vi "requestStatus.vi"(8 "error in (no error)":errorcluster, 11 "MonoClientCommunicator in":refnum<class "MonoClientCommunicator.lvclass">) -> (0 "error out":errorcluster, 2 "DeviceStatus":T1, 3 "MonoClientCommunicator out":refnum<class "MonoClientCommunicator.lvclass">)   [LabVIEW 2016, in "MonoClientCommunicator.lvclass"]
uses:
  MonoClientCommunicator.lvclass
  Typedefs/DeviceStatus.ctl
  Typedefs/MonoCommand.ctl
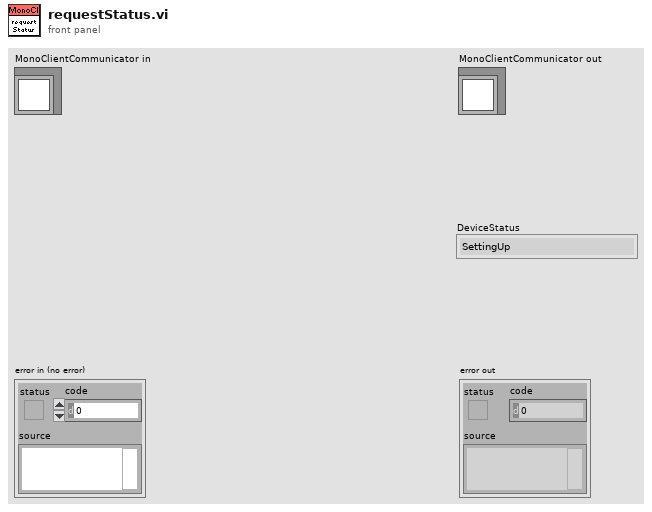
[diagram p1: front panel]
types:
  T1 = typedef "DeviceStatus.ctl" = enum16{"SettingUp", "Ready", "Offline", "Fault"}
  T2 = typedef "MonoCommand.ctl" = enum16{"getGrating", "getFrontEntranceSlitPosition", "getFrontExitSlitPosition", "getWavelength", "setWavelength", "setGrating", "setFrontEntranceSlitPosition", "setFrontExitSlitPosition", "calibrateWavelength", "getStatus", "Unknown", "reset", "setAll"}
  T3 = typedef "publishers.ctl" = enum16{"Wavelength", "Grating", "FrontEntranceSlitPosition", "FrontExitSlitPosition", "SoftwareStatus", "MonochromatorId", "Ack"}
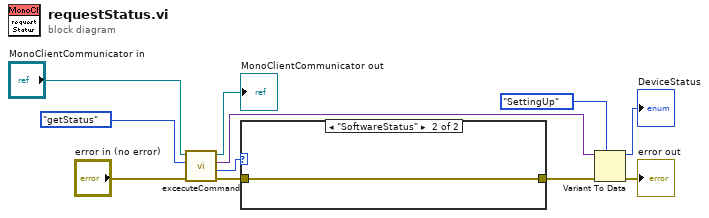
[diagram p0: block diagram]
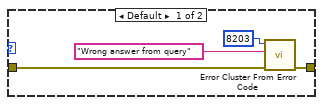
[diagram p2: hidden frame]
diagram:
  n1 = call "excecuteCommand.vi"("error in (no error)"="error in (no error)", "MonoCommand"=MonoCommand."getStatus", "MonoClientCommunicator in"="MonoClientCommunicator in") -> ("error out"=w8:errorcluster, "parameter"=w3:T3, "value"=w4:variant, "MonoClientCommunicator out"=→"MonoClientCommunicator out":refnum<class "MonoClientCommunicator.lvclass">)  [unwired: 5 in]
  n2 = case shown="\"SoftwareStatus\"" w3 {
    tunnel: w8 -> [w13 w16]
    tunnel: [w12 w16] -> w9
    frame Default {
      n3 = call <vilib>:"Error Cluster From Error Code.vi"("error in (no error)"=w13, "error message (\"\")"="Wrong answer from query" ("error message (\"\")"), "error code (0)"=8203) -> ("error out"=w12:errorcluster)  [unwired: 6 in]
    }
    frame "SoftwareStatus" {
    }
  }
  n4 = Variant To Data(error in=w9, type=DeviceStatus."SettingUp" ("DeviceStatus"), Variant=w4) -> (data=→"DeviceStatus":T1, error out=→"error out":errorcluster)
